vi "运维调试_挥发酚.vi"() -> ()   [LabVIEW 2016, in "挥发酚.lvlib"]
uses:
  <vilib>/Utility/miscctls.llb/LVPointTypeDef.ctl
  <vilib>/ptbypt/NI_PtbyPt.lvlib
panel:
  out "当前步骤:":string
  in  "告警代码":u16
  in  "周期设置":bool
  out "权限等级":string
  in  "参数查询":bool
  in  "平台反控标样校准":enum16{"标液1", "标液2", "标液3"}(ring)
  in  "平台反控校准量程":enum16{"低量程1", "低量程2", "高量程1", "高量程2"}(ring)
  in  "返回 3":bool
  in  "返回 2":bool
  out "单位:":T1(ring)
  out "运行状态":T2 {"数据时间:" format="%<%y/%m/%d %H:%M:%S>T"; "仪器时间:" format="%<%y/%m/%d %H:%M:%S>T"}
  out "模块版本号":string
  in  "布尔":bool
  out "字符串":string
  in  "返回":bool
  in  "设置":bool
  out "集成报警信息":string
  in  "停止":bool
  in  "手动启动":bool
  # "."
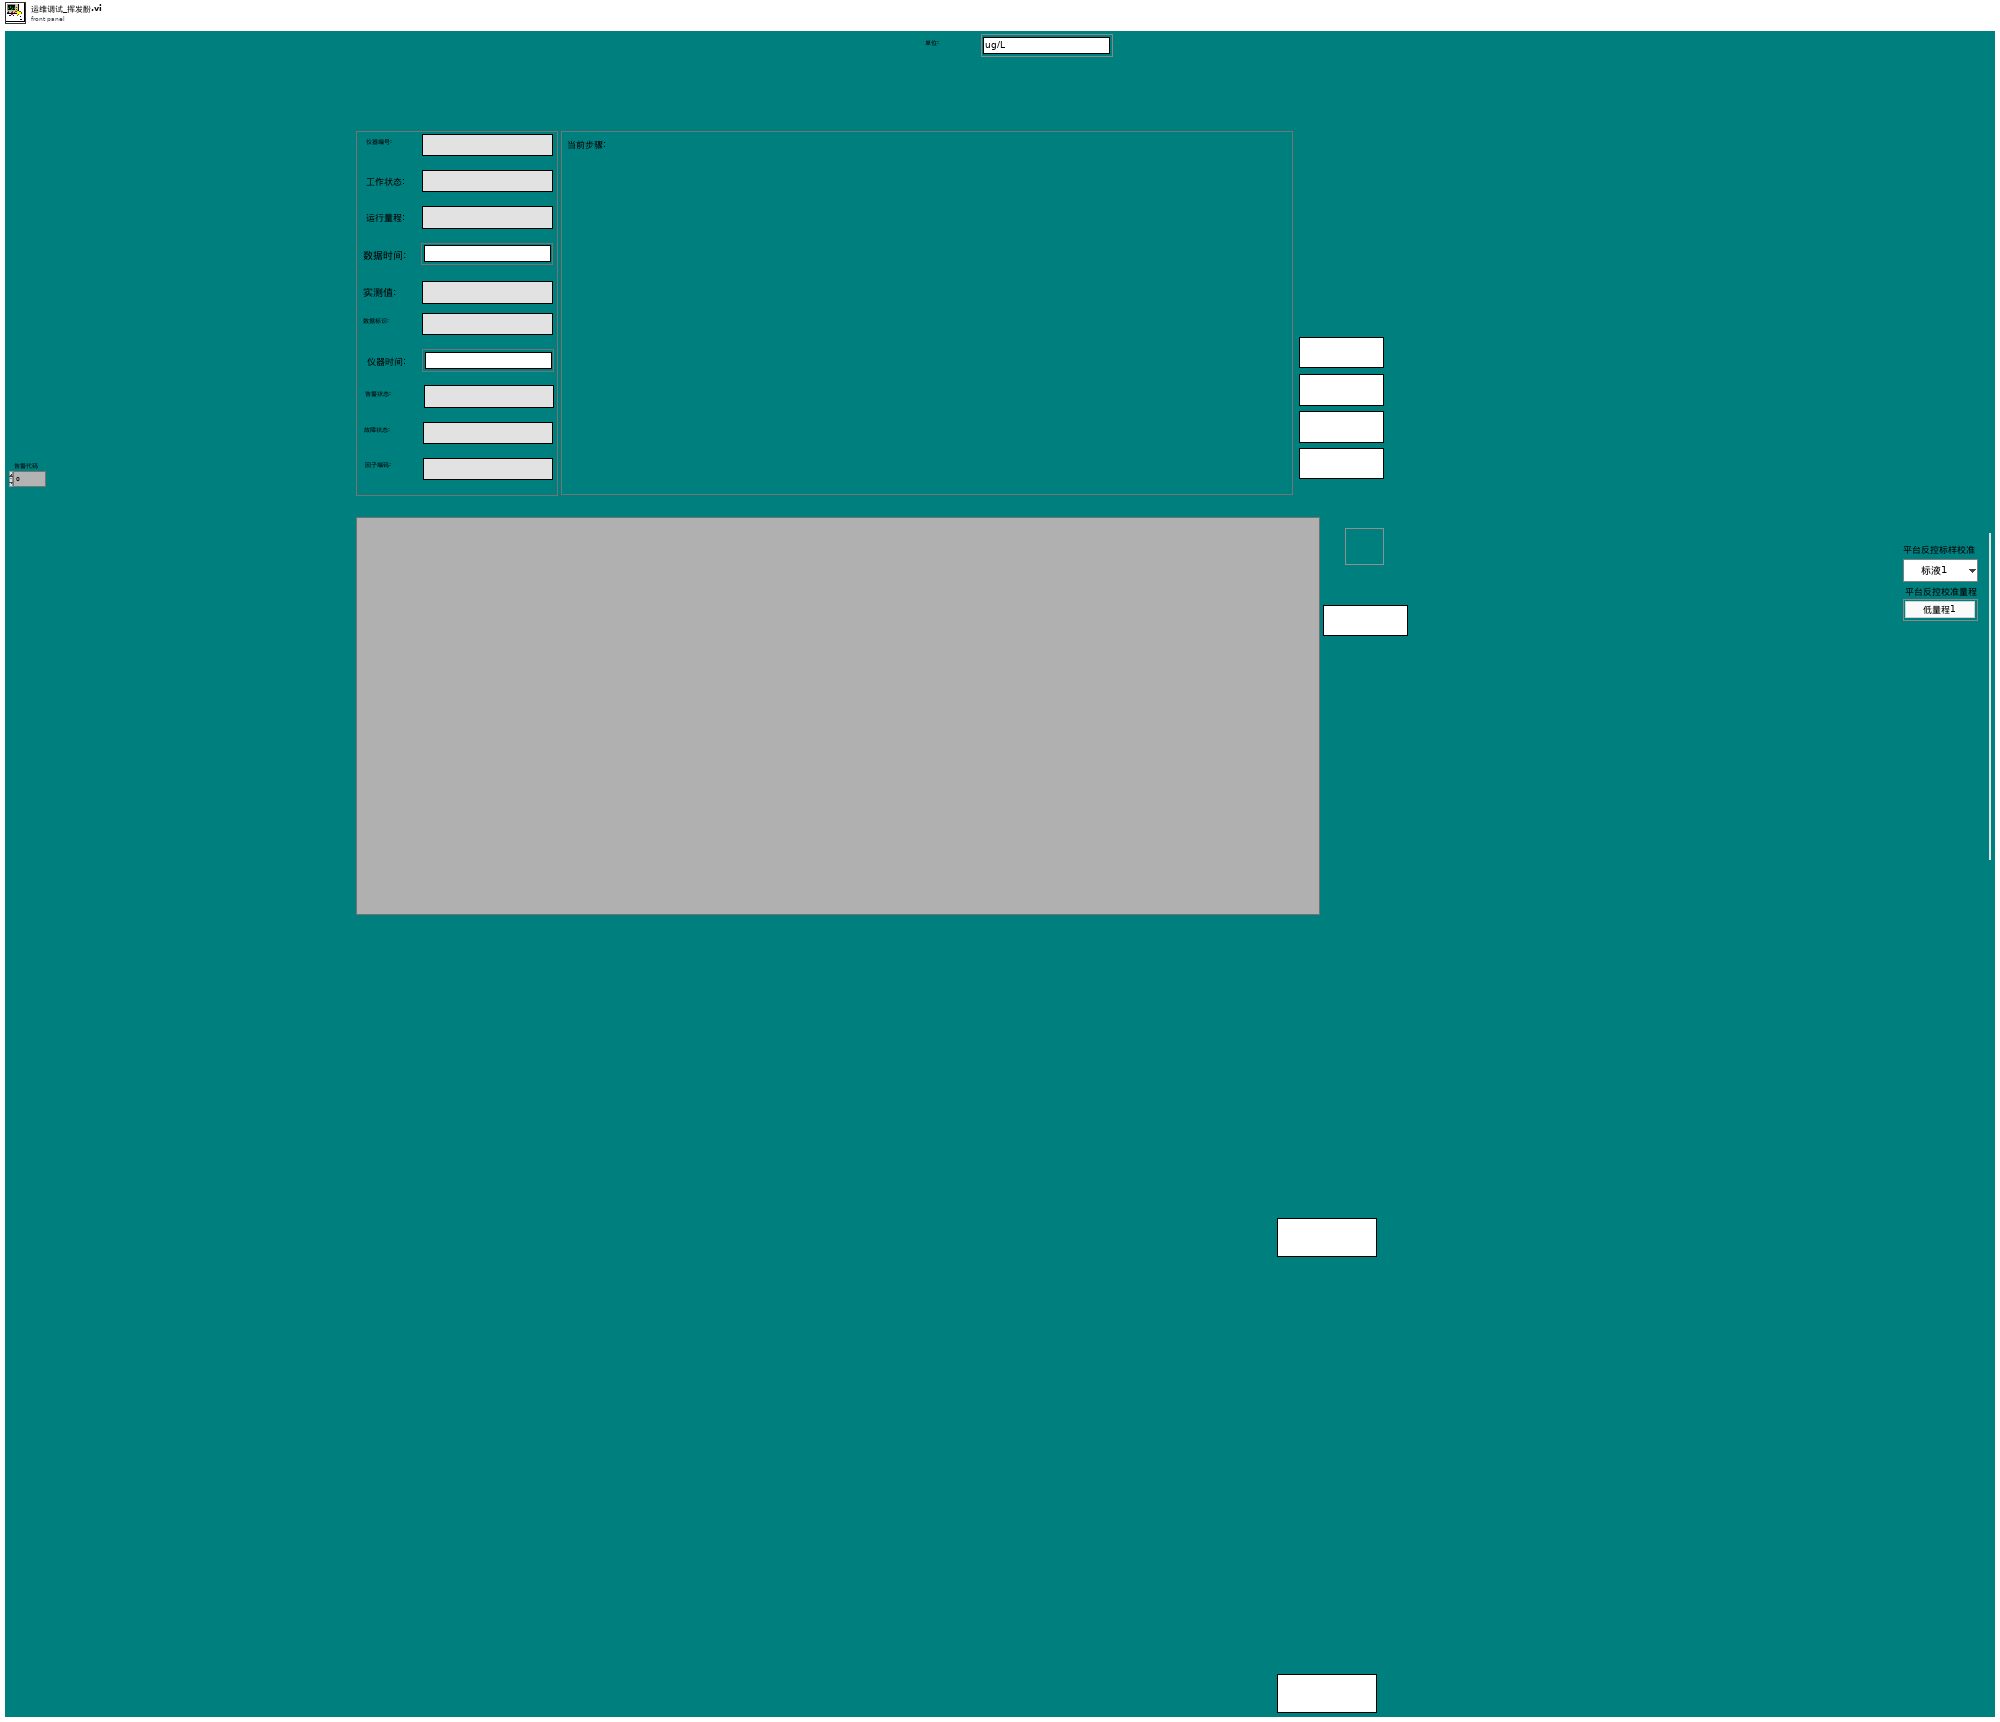
[diagram p1: front panel]
types:
  T1 = enum16{"ug/L", "mg/L", "ppm", "mg/m3", "cm", "ppb", "ug/m3", "%", "nmol/mol", "umol/mol", "MPN/L", "MPN/100ml", "ng/m3", "NTU", "无量纲", "ms/cm", "us/cm", "℃", "mV", "万个/L"}
  T2 = cluster{"仪器编号:":string, "工作状态:":string, "运行量程: ":string, "数据时间:":timestamp, "实测值:":string, "数据标识: ":string, "仪器时间:":timestamp, "告警状态: ":string, "故障状态:  ":string, "因子编码:":string}
  T3 = cluster{"Major":u16, "Minor":u16, "Fix":u16, "Build":u16}
  T4 = typedef "LVPointTypeDef.ctl" = cluster{"Horizontal":i16, "Vertical":i16}
  T5 = cluster{"因子编码":u32, "单位":u16, "标样2参考值":sgl, "水样数据时间":timestamp, "水样实测值":sgl, "水样数据标识":string, "标样2数据时间":timestamp, "标样2实测值":sgl, "标样2数据标识":string, "空白数据时间":timestamp, "空白实测值":sgl, "空白数据标识":string, "零点核查数据时间":timestamp, "零点核查实测值":sgl, "零点核查数据标识":string, "跨度核查数据时间":timestamp, "跨度核查实测值":sgl, "跨度核查数据标识":string, "加标回收数据时间":timestamp, "加标回收实测值":sgl, "加标回收数据标识":string, "平行样数据时间":timestamp, "平行样实测值":sgl, "平行样数据标识":string, "标样1参考值":sgl, "标样1数据时间":timestamp, "标样1实测值":sgl, "标样1数据标识":string, "标样核查数据时间":timestamp, "标样核查实测值":sgl, "标样核查数据标识":string}
  T6 = cluster{"系统时间":timestamp, "工作状态":u16, "测量模式":enum16{"待机", "连续模式", "周期模式", "定点模式", "受控模式", "手动模式"}, "告警代码":u16, "故障代码":u16, "日志代码":u16, "软件版本":u16, "测量间隔":u16, "消解实时温度":dbl, "校准间隔（天）":u16, "校准间隔（时）":u16, "周期测量时间（23_16）":u16, "周期测量时间（15_0）":u16, "清洗周期（次数）":u16, "运行模式":u16, "自动校准状态":u16, "自动清洗状态":u16}
  T7 = cluster{"测量精度":u16, "消解温度":u16, "消解时长":u16, "量程下限":sgl, "量程上限":sgl, "曲线斜率K":sgl, "曲线斜率B":sgl, "标定日期":timestamp, "标液1浓度":sgl, "标液1测量过程值":sgl, "标液2浓度":sgl, "标液2测量过程值":sgl, "标液3浓度":sgl, "标液3测量过程值":sgl, "标液4浓度":sgl, "标液4测量过程值":sgl, "标液5浓度":sgl, "标液5测量过程值":sgl, "线性相关系数":sgl, "试剂余量":u32, "测量滴定值或吸光度":sgl, "标样2校准时间":timestamp, "检出限值":sgl, "校准系数":sgl, "设备系列号":string, "显色温度":u16, "显色时间":u16, "试剂余量1":u16, "试剂余量2":u16, "试剂余量3":u16, "试剂余量4":u16, "试剂余量5":u16, "试剂余量6":u16, "试剂余量7":u16, "试剂余量8":u16, "试剂余量9":u16, "试剂余量10":u16, "当前量程低位":sgl, "当前量程高位":sgl}
  T8 = typedef "Alarm interface.lvlib/报警短信语音交互.ctl" = cluster{"参数":string, "元器件":string, "故障现象":string, "code":string, "platform_alarm_code":string, "solutionList":cluster{"reason":string, "solution":string}[]}
  T9 = enum8{"Enabled", "Disabled", "Disabled and Grayed Out"}
  T10 = enum32{"Bad", "Idle", "Run top level", "Running"}
  T11 = enum16{"空闲", "水样测试", "标样核查", "零点核查", "跨度核查", "空白测试", "平行样测试", "加标回收", "空白校准", "标样校准", "初始化（清洗）"}
  T12 = typedef "TimingControl.lvlib/TimingControl.lvclass/国标控制命令.ctl" = enum16{"启动测量", "标样核查", "零点核查", "跨度核查", "空白测试", "平行样测试", "加标回收", "空白校准", "标样校准", "初始化（清洗）", "停止测试", "仪器重启", "校时", "模式设置", "测量间隔设置"}
  T13 = typedef "TimingControl.lvlib/TimingControl.lvclass/测量参数.ctl" = u16
  T14 = cluster{"时间标识":timestamp, "设备":string, "日志信息":string, "流程参数":string}
  T15 = cluster{"水样数据时间":timestamp, "空白数据时间":timestamp, "零点核查数据时间":timestamp, "跨度核查数据时间":timestamp, "加标回收数据时间":timestamp, "平行样数据时间":timestamp, "标样核查数据时间":timestamp, "标样1数据时间":timestamp, "标样2数据时间":timestamp}
  T16 = cluster{"站号":u16, "量程切换":enum32{"H", "L", "AUTO"}, "控制命令":u16, "模式设置":enum16{"待机", "连续模式", "周期模式", "定点模式", "受控模式", "手动模式"}, "测量间隔":u16}
  T17 = cluster{"跨度值":dbl, "零点标准液浓度":dbl, "跨度标准液浓度":dbl, "标准液标准浓度":dbl, "零点标准液偏差":dbl, "跨度标准液偏差":dbl, "标准液标准偏差":dbl}
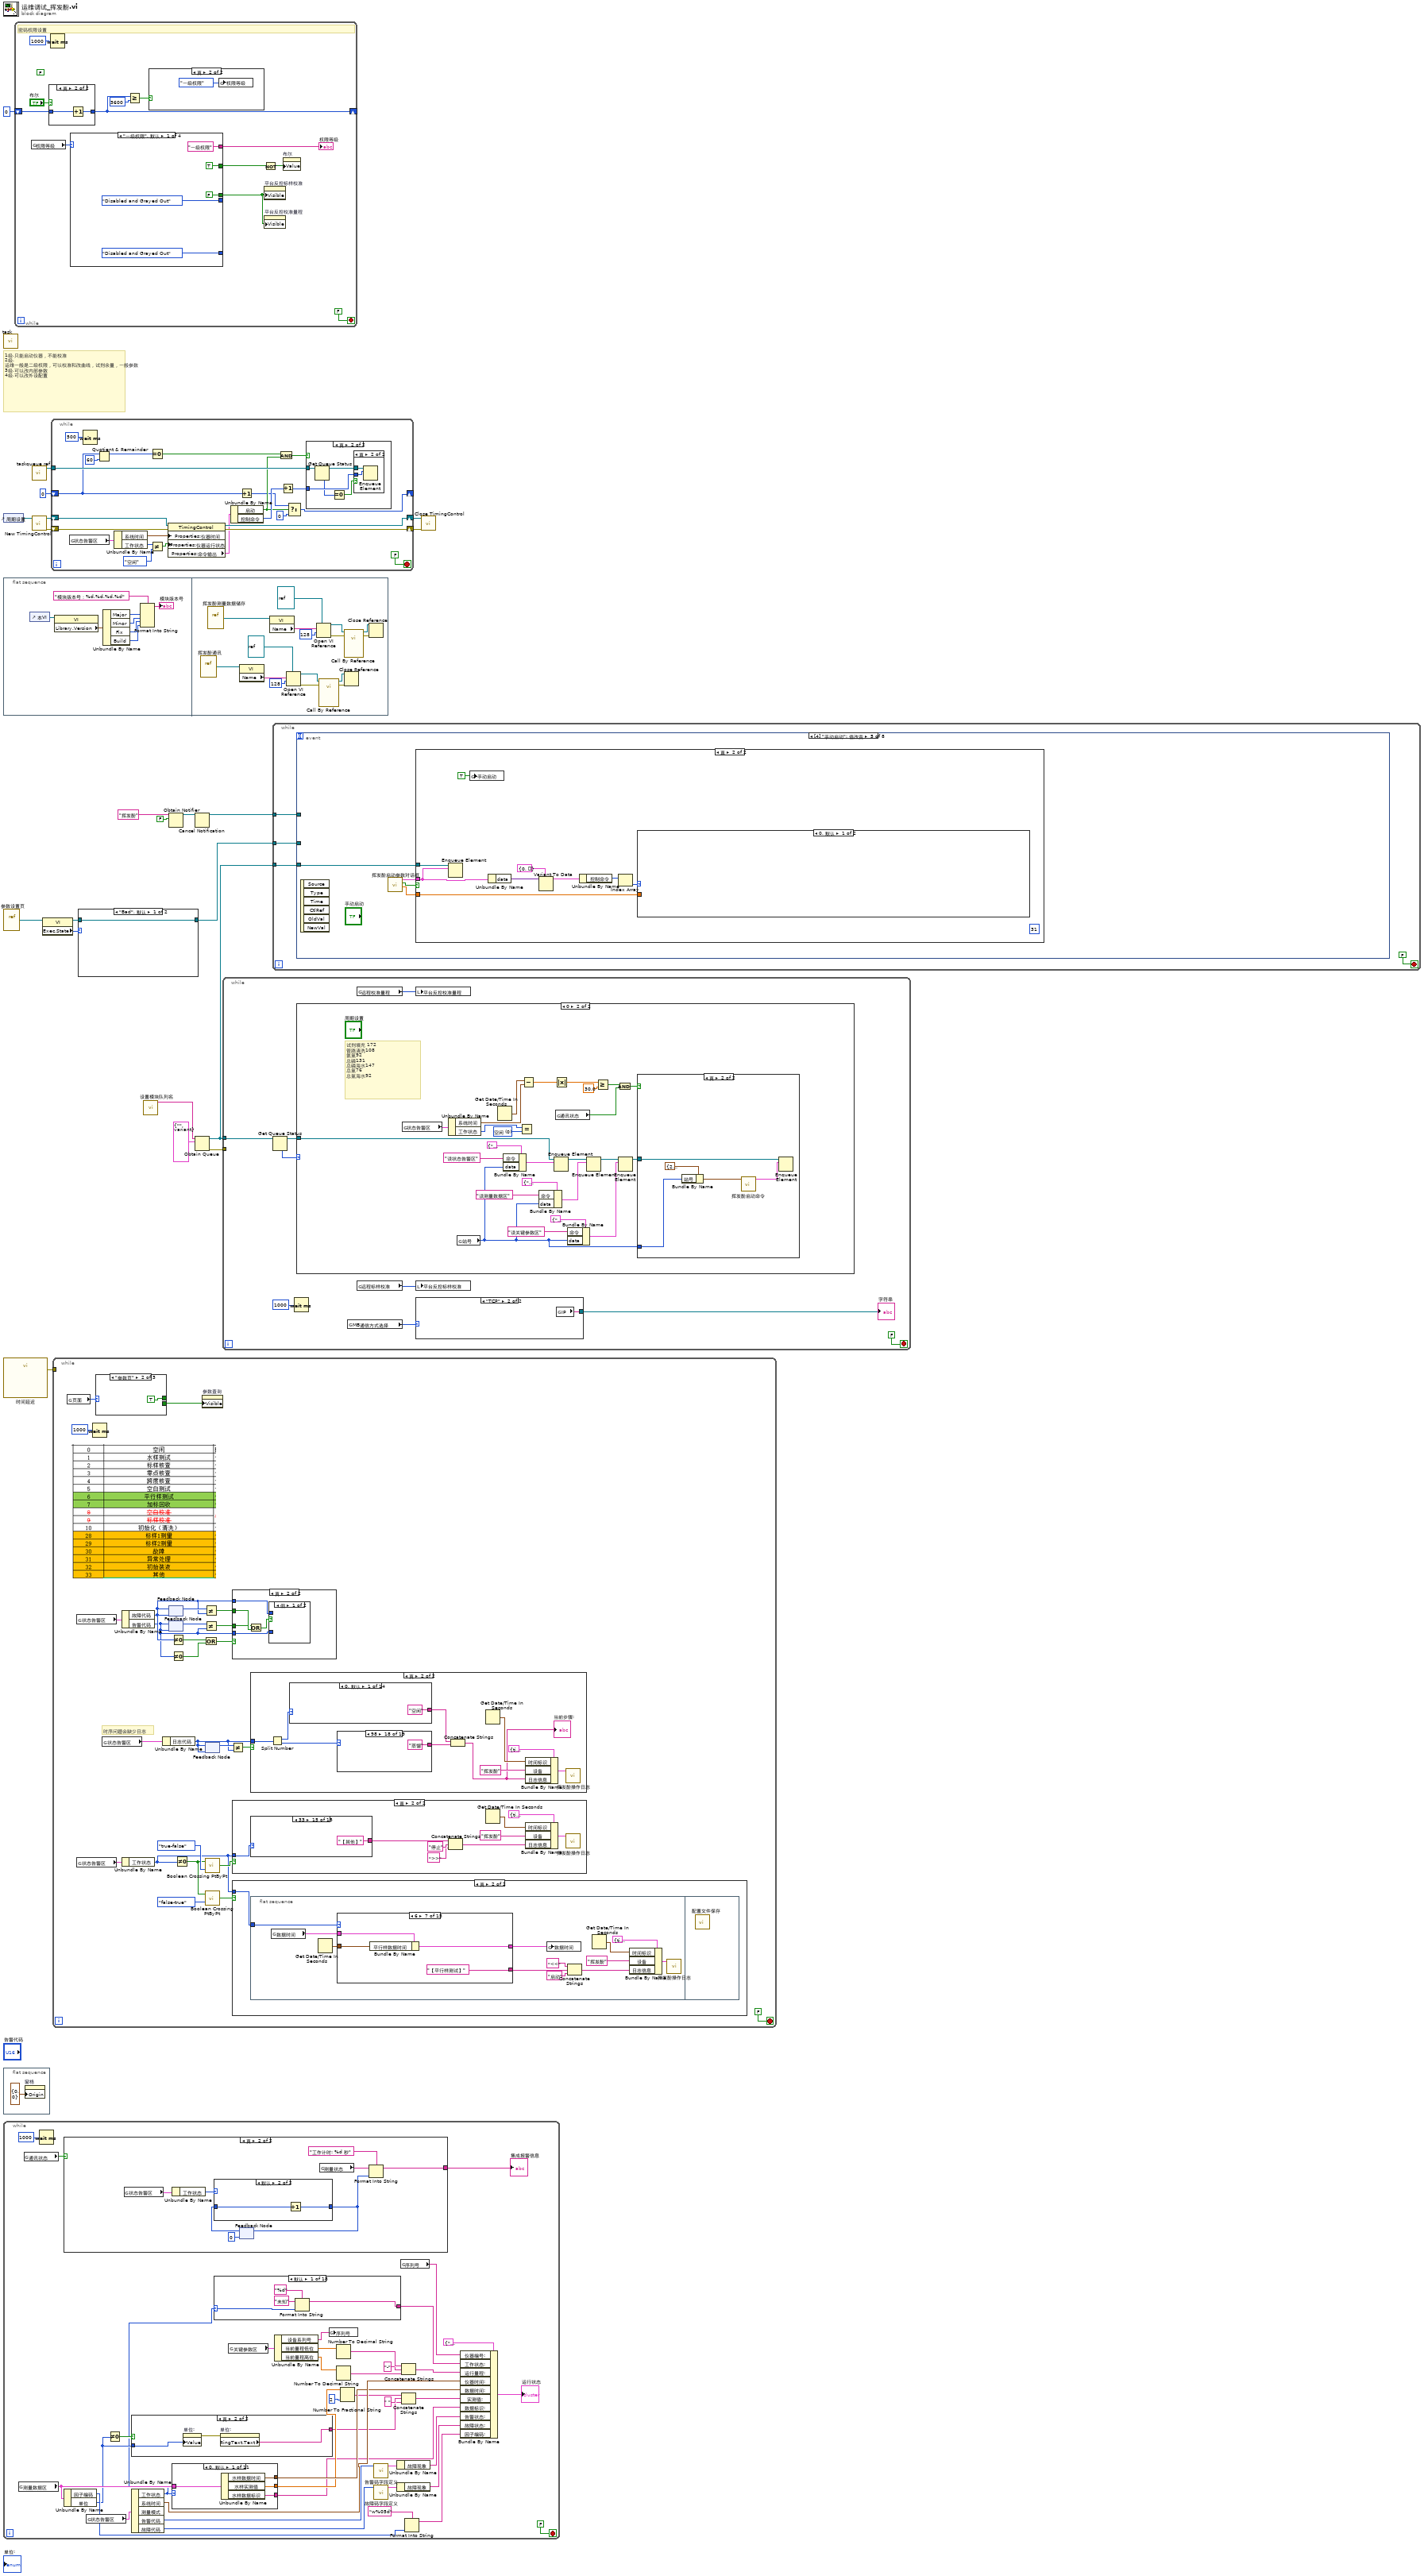
[diagram p0: block diagram]
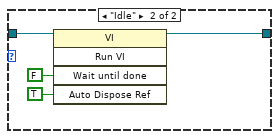
[diagram p2: hidden frame]
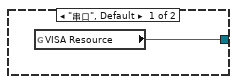
[diagram p5: hidden frame]
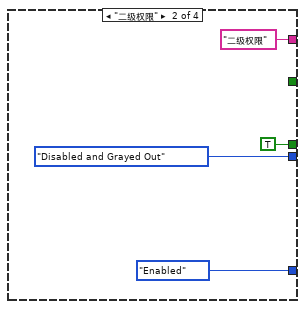
[diagram p8: hidden frame]
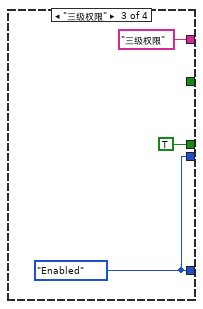
[diagram p9: hidden frame]
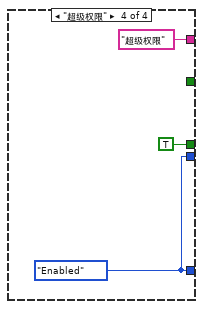
[diagram p10: hidden frame]
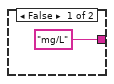
[diagram p13: hidden frame]
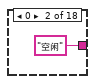
[diagram p14: hidden frame]
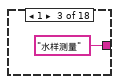
[diagram p15: hidden frame]
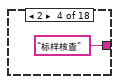
[diagram p16: hidden frame]
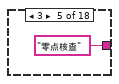
[diagram p17: hidden frame]
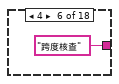
[diagram p18: hidden frame]
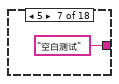
[diagram p19: hidden frame]
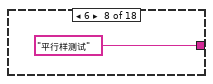
[diagram p20: hidden frame]
diagram:
  # "1级.只能启动仪器，不能校准\n2级.运维一般是二级权限，可以校准和改曲线，试剂余量，一般参数\n3级.可以改内部参数\n4级.可以改外设配置"
  n1 = call "task.vi"() -> ()  [unwired: 12 in]
  n2 = control-ref of="周期设置"() -> (w5:refnum<vi>)
  n3 = flat-sequence {
    frame #0 {
      n4 = control-ref of="本VI"() -> (w29:refnum<vi>)
      n5 = property class="VI"(reference=w29) -> ("Library.Version"=w28:T3)  [unwired: 1 in, 2 out]
      n6 = Unbundle By Name(w28) -> ("Major"=w26:u16, "Minor"=w25:u16, "Fix"=w24:u16, "Build"=w23:u16)
      n7 = Format Into String(format string="模块版本号：%d.%d.%d.%d" ("格式字符串"), w26, w25, w24, w23) -> (resulting string=→"模块版本号":string)  [unwired: 2 in, 1 out]
    }
    frame #1 {
      n8 = vi-ref "挥发酚通讯.vi"() -> (w37:refnum<vi>)
      n9 = vi-ref "挥发酚测量数据储存.vi"() -> (w45:refnum<vi>)
      n10 = property class="VI"(reference=w37) -> ("Name"=w36:string)  [unwired: 1 in, 2 out]
      n11 = property class="VI"(reference=w45) -> ("Name"=w38:string)  [unwired: 1 in, 2 out]
      n12 = Open VI Reference(type specifier VI Refnum (for type only)=refnum<vi> refnum, vi path=w36, options=128 ("选项")) -> (vi reference=w34:refnum<vi>, error out=w32:errorcluster)  [unwired: 3 in]
      n13 = Open VI Reference(type specifier VI Refnum (for type only)=refnum<vi> refnum, vi path=w38, options=128 ("选项")) -> (vi reference=w40:refnum<vi>, error out=w42:errorcluster)  [unwired: 3 in]
      n14 = call-by-ref "?"(reference=w34, error in=w32) -> (reference out=w30:refnum<vi>, error out=w31:errorcluster)  [unwired: 12 in]
      n15 = call-by-ref "?"(reference=w40, error in=w42) -> (reference out=w44:refnum<vi>, error out=w43:errorcluster)  [unwired: 12 in]
      n16 = Close Reference(reference=w30, error in (no error)=w31) -> ()  [unwired: 1 out]
      n17 = Close Reference(reference=w44, error in (no error)=w43) -> ()  [unwired: 1 out]
    }
  }
  n18 = vi-ref "参数设置页.vi"() -> (w12:refnum<vi>)
  n19 = call "时间延迟"() -> ("error out"=w19:errorcluster)  [unwired: 11 in]
  n20 = flat-sequence {
    frame #0 {
      n21 = property on="窗格" class="Pane"("Origin"=T4 {"Horizontal"=0, "Vertical"=0} ("原点")) -> ()  [unwired: 2 in, 2 out]
    }
  }
  n22 = while {
    stop <- FALSE stop-if-true
    n23 = global read "VAR挥发酚全局变量.vi" "测量数据区"() -> (w80:T5)
    n24 = global read "VAR挥发酚全局变量.vi" "通讯状态"() -> (w83:bool)
    n25 = Wait (ms)(milliseconds to wait=u32 1000 ("等待时间（毫秒）")) -> ()  [unwired: 1 out]
    n26 = case shown="真" w83 {
      tunnel: ["通讯异常" ("集成报警信息") w157] -> w82
      frame False {
      }
      frame True {
        n27 = global read "VAR挥发酚全局变量.vi" "状态告警区"() -> (w163:T6)
        n28 = Unbundle By Name(w163) -> ("工作状态"=w162:u16)
        n29 = feedback #1(0) -> (w160:i32)
        n30 = case shown="默认" w162 {
          tunnel: w160 -> [_ w165]
          tunnel: [_ w164] -> w158
          frame 0 {
          }
          frame Default {
            n31 = Increment(x=w165) -> (x+1=w164:i32)
          }
        }
        n32 = feedback-in #1(w158) -> ()
        n33 = global read "VAR挥发酚全局变量.vi" "测量状态"() -> (w156:string)
        n34 = Format Into String(format string="工作计时: %d 秒" ("格式字符串"), initial string=w156, w158) -> (resulting string=w157:string)  [unwired: 1 in, 1 out]
      }
    }
    "集成报警信息" <- w82
    n35 = Unbundle By Name(w80) -> ("因子编码"=w63:u32, "单位"=w60:u16)
    n36 = global read "VAR挥发酚全局变量.vi" "状态告警区"() -> (w81:T6)
    n37 = Not Equal To 0?(x=w60) -> (x != 0?=w61:bool)
    n38 = case shown="真" w61 {
      tunnel: ["mg/L" ("RingText.Text") w88] -> w65
      tunnel: w60 -> [_ w87]
      frame False {
      }
      frame True {
        n39 = property on="单位:" class="Enum (严格)"("Value"=w87) -> (error out=w89:errorcluster)  [unwired: 2 in, 1 out]
        n40 = property on="单位:" class="Enum (严格)"(error in=w89) -> ("RingText.Text"=w88:string)  [unwired: 1 in, 2 out]
      }
    }
    n41 = Unbundle By Name(w81) -> ("工作状态"=w55:u16, "系统时间"=w77:timestamp, "告警代码"=w67:u16, "故障代码"=w66:u16)  [unwired: 1 out]
    n42 = case shown="0, 默认" w55 {
      tunnel: [w114 w118 w122 w126 w130 w134 w138 w142 w145 w149 w154] -> w74
      tunnel: [w112 w117 w121 w125 w129 w133 w136 w141 w144 w148 w153] -> w69
      tunnel: [w111 w116 w120 w124 w128 w132 w135 w140 w143 w147 w152] -> w68
      tunnel: w80 -> [w113 w115 w119 w123 w127 w131 w137 w139 w146 w150 w151]
      frame 0, Default {
        n43 = Unbundle By Name(w113) -> ("水样数据时间"=w114:timestamp, "水样实测值"=w112:sgl, "水样数据标识"=w111:string)
      }
      frame 1 {
        n44 = Unbundle By Name(w115) -> ("水样数据时间"=w118:timestamp, "水样实测值"=w117:sgl, "水样数据标识"=w116:string)
      }
      frame 2 {
        n45 = Unbundle By Name(w119) -> ("标样核查数据时间"=w122:timestamp, "标样核查实测值"=w121:sgl, "标样核查数据标识"=w120:string)
      }
      frame 3 {
        n46 = Unbundle By Name(w123) -> ("零点核查数据时间"=w126:timestamp, "零点核查实测值"=w125:sgl, "零点核查数据标识"=w124:string)
      }
      frame 4 {
        n47 = Unbundle By Name(w127) -> ("跨度核查数据时间"=w130:timestamp, "跨度核查实测值"=w129:sgl, "跨度核查数据标识"=w128:string)
      }
      frame 5 {
        n48 = Unbundle By Name(w131) -> ("空白数据时间"=w134:timestamp, "空白实测值"=w133:sgl, "空白数据标识"=w132:string)
      }
      frame 6 {
        n49 = Unbundle By Name(w137) -> ("平行样数据时间"=w138:timestamp, "平行样实测值"=w136:sgl, "平行样数据标识"=w135:string)
      }
      frame 7 {
        n50 = Unbundle By Name(w139) -> ("加标回收数据时间"=w142:timestamp, "加标回收实测值"=w141:sgl, "加标回收数据标识"=w140:string)
      }
      frame 28 {
        n51 = Unbundle By Name(w146) -> ("标样1数据时间"=w145:timestamp, "标样1实测值"=w144:sgl, "标样1数据标识"=w143:string)
      }
      frame 29 {
        n52 = Unbundle By Name(w150) -> ("标样2数据时间"=w149:timestamp, "标样2实测值"=w148:sgl, "标样2数据标识"=w147:string)
      }
      frame 10 {
        n53 = Unbundle By Name(w151) -> ("水样数据时间"=w154:timestamp, "水样实测值"=w153:sgl, "水样数据标识"=w152:string)
      }
    }
    n54 = case shown="默认" w55 {
      selector: w55 -> [w90 _ _ _ _ _ _ _ _ _ _ _ _ _ _ _ _ _]
      tunnel: [w91 "空闲" ("工作状态") "水样测量" ("工作状态") "标样核查" ("工作状态") "零点核查" ("工作状态") "跨度核查" ("工作状态") "空白测试" ("工作状态") "平行样测试" ("工作状态") "加标回收" ("工作状态") "空白校准" ("工作状态") "标样校准" ("工作状态") "初始化" ("工作状态") "标样1测量" ("工作状态") "标样2测量" ("工作状态") "故障" ("工作状态") "异常处理" ("工作状态") "初始装液" ("工作状态") "其他" ("工作状态")] -> w78
      frame Default {
        n55 = Format Into String(format string="%d" ("格式字符串"), initial string="未知" ("工作状态"), w90) -> (resulting string=w91:string)  [unwired: 1 in, 1 out]
      }
      frame 0 {
      }
      frame 1 {
      }
      frame 2 {
      }
      frame 3 {
      }
      frame 4 {
      }
      frame 5 {
      }
      frame 6 {
      }
      frame 7 {
      }
      frame 8 {
      }
      frame 9 {
      }
      frame 10 {
      }
      frame 28 {
      }
      frame 29 {
      }
      frame 30 {
      }
      frame 31 {
      }
      frame 32 {
      }
      frame 33 {
      }
    }
    n56 = global read "VAR挥发酚全局变量.vi" "关键参数区"() -> (w54:T7)
    n57 = Unbundle By Name(w54) -> ("设备系列号"=w53:string, "当前量程低位"=w52:sgl, "当前量程高位"=w49:sgl)
    n58 = global write "VAR挥发酚全局变量.vi" "序列号"(w53) -> ()
    n59 = Number To Decimal String(number=w52) -> (decimal integer string=w51:string)  [unwired: 1 in]
    n60 = Number To Decimal String(number=w49) -> (decimal integer string=w48:string)  [unwired: 1 in]
    n61 = Number To Fractional String(number=w69, precision (6)=i16 2 ("精度(6)")) -> (F-format string=w72:string)  [unwired: 2 in]
    n62 = call "告警码字段定义.vi"("告警代码"=w67) -> ("data"=w59:T8)  [unwired: 10 in]
    n63 = call "故障码字段定义.vi"("故障代码"=w66) -> ("data"=w58:T8)  [unwired: 10 in]
    n64 = Unbundle By Name(w59) -> ("故障现象"=w56:string)
    n65 = Unbundle By Name(w58) -> ("故障现象"=w57:string)
    n66 = global read "VAR挥发酚全局变量.vi" "序列号"() -> (w79:string)
    n67 = Concatenate Strings(w51, "-" ("字符串"), w48) -> (w47:string)
    n68 = Concatenate Strings(w72, " " ("字符串"), w65) -> (w70:string)
    n69 = Format Into String(format string="w%05d" ("格式字符串"), w63) -> (resulting string=w62:string)  [unwired: 2 in, 1 out]
    n70 = Bundle By Name(cluster=T2 {"仪器编号:"="", "工作状态:"="", "运行量程: "="", "数据时间:"=timestamp(0 s since 1904-01-01), "实测值:"="", "数据标识: "="", "仪器时间:"=timestamp(0 s since 1904-01-01), "告警状态: "="", "故障状态:  "="", "因子编码:"=""} ("运行状态"), "仪器编号:"=w79, "工作状态:"=w78, "运行量程:"=w47, "仪器时间:"=w77, "数据时间:"=w74, "实测值:"=w70, "数据标识:"=w68, "告警状态:"=w56, "故障状态:"=w57, "因子编码:"=w62) -> (→"运行状态":T2)
  }
  n71 = while {
    shift-right: [w174] -> _
    shift-left: u32 0 ("等待时间（毫秒）") -> [w175]
    stop <- FALSE stop-if-true
    (unwired) FALSE ("可见")
    # "密码权限设置"
    n72 = global read "VAR挥发酚全局变量.vi" "权限等级"() -> (w171:enum16{"一级权限", "二级权限", "三级权限", "超级权限"})
    n73 = case shown="真" "布尔" {
      tunnel: w175 -> [_ w195]
      tunnel: [_ w194] -> w174
      frame False {
      }
      frame True {
        n74 = Increment(x=w195) -> (x+1=w194:u32)
      }
    }
    n75 = Wait (ms)(milliseconds to wait=u32 1000 ("等待时间（毫秒）")) -> ()  [unwired: 1 out]
    n76 = case shown="\"一级权限\", 默认" w171 {
      tunnel: [T9."Disabled and Grayed Out" ("f") T9."Enabled" ("禁用") w189 w192] -> _
      tunnel: [T9."Disabled and Grayed Out" ("f") T9."Disabled and Grayed Out" ("f") w189 w192] -> _
      tunnel: [FALSE ("可见") TRUE ("可见") TRUE ("可见") TRUE ("可见")] -> w170
      tunnel: ["一级权限" "二级权限" "三级权限" "超级权限"] -> w169
      tunnel: [TRUE _ _ _] -> w168
      frame "一级权限", Default {
      }
      frame "二级权限" {
      }
      frame "三级权限" {
        w189 = T9."Enabled" ("禁用")
      }
      frame "超级权限" {
        w192 = T9."Enabled" ("禁用")
      }
    }
    "权限等级" <- w169
    n77 = Greater Or Equal?(x=w174, y=u32 3600) -> (x >= y?=w172:bool)
    n78 = case shown="真" w172 {
      frame False {
      }
      frame True {
        n79 = global write "VAR挥发酚全局变量.vi" "权限等级"(enum16{"一级权限", "二级权限", "三级权限", "超级权限"}."一级权限" ("权限等级")) -> ()
      }
    }
    n80 = Not(x=w168) -> (.not. x?=w166:bool)
    n81 = property on="平台反控标样校准" class="Enum (严格)"("Visible"=w170) -> ()  [unwired: 2 in, 2 out]
    n82 = property on="平台反控校准量程" class="Enum (严格)"("Visible"=w170) -> ()  [unwired: 2 in, 2 out]
    n83 = property on="布尔" class="Bool (严格)"("Value"=w166) -> ()  [unwired: 2 in, 2 out]
  }
  n84 = call "taskqueue ref.vi"() -> ("队列输出"=w8:refnum<queue>)  [unwired: 10 in, 1 out]
  n85 = call "New TimingControl.vi"("Reference"=w5) -> ("error out"=w3:errorcluster, "TimingControl out"=w4:refnum<class "TimingControl.lvclass">)  [unwired: 9 in]
  n86 = property class="VI"(reference=w12) -> (reference out=w10:refnum<vi>, "Exec.State"=w11:T10)  [unwired: 1 in, 1 out]
  n87 = while {
    tunnel: w8 -> [w215]
    shift-right: [w205] -> _
    shift-left: u32 0 ("等待时间（毫秒）") -> [w206]
    shift-right: [w200] -> w2
    shift-left: w4 -> [w202]
    shift-right: [w199] -> w1
    shift-left: w3 -> [w201]
    stop <- FALSE stop-if-true
    n88 = global read "VAR挥发酚全局变量.vi" "状态告警区"() -> (w217:T6)
    n89 = Wait (ms)(milliseconds to wait=u32 500 ("等待时间（毫秒）")) -> ()  [unwired: 1 out]
    n90 = Quotient & Remainder(x=w206, y=u32 60) -> (x-y*floor(x/y)=w203:u32)  [unwired: 1 out]
    n91 = Unbundle By Name(w217) -> ("系统时间"=w197:timestamp, "工作状态"=w210:u16)
    n92 = Equal To 0?(x=w203) -> (x = 0?=w212:bool)
    n93 = Not Equal?(x=w210, y=T11."空闲") -> (x != y?=w196:bool)
    n94 = property class="TimingControl"(reference=w202, error in=w201, "Properties:仪器时间"=w197, "Properties:仪器运行状态"=w196) -> (reference out=w200:refnum<class "TimingControl.lvclass">, error out=w199:errorcluster, "Properties:命令输出"=w198:cluster{"启动":bool, "控制命令":T12, "测量参数":T13})
    n95 = Unbundle By Name(w198) -> ("启动"=w209:bool, "控制命令"=w214:T12)
    n96 = Increment(x=w206) -> (x+1=w208:u32)
    n97 = And(x=w212, y=w209) -> (x .and. y?=w211:bool)
    n98 = Increment(x=w214) -> (x+1=w213:T12)
    n99 = Select(t=w208, s=w209, f=u32 0) -> (s? t:f=w205:u32)
    n100 = case shown="真" w211 {
      tunnel: w215 -> [_ w224]
      tunnel: w213 -> [_ w223]
      frame False {
      }
      frame True {
        n101 = Get Queue Status(queue=w224) -> (queue out=w222:refnum<queue>, # elements in queue=w221:i32)  [unwired: 2 in, 6 out]
        n102 = Equal To 0?(x=w221) -> (x = 0?=w220:bool)
        n103 = case shown="真" w220 {
          tunnel: w223 -> [_ w226]
          tunnel: w222 -> [_ w225]
          frame False {
          }
          frame True {
            n104 = Enqueue Element(queue=w225, element=w226) -> ()  [unwired: 2 in, 3 out]
          }
        }
      }
    }
  }
  n105 = while {
    tunnel: w19 -> [_]
    stop <- FALSE stop-if-true
    # "时序问题会缺少日志"
    n106 = global read "VAR挥发酚全局变量.vi" "页面"() -> (w232:enum16{"主页", "参数页", "校准页"})
    n107 = global read "VAR挥发酚全局变量.vi" "状态告警区"() -> (w249:T6)
    n108 = global read "VAR挥发酚全局变量.vi" "状态告警区"() -> (w246:T6)
    n109 = Wait (ms)(milliseconds to wait=u32 1000 ("等待时间（毫秒）")) -> ()  [unwired: 1 out]
    n110 = case shown="\"参数页\"" w232 {
      tunnel: [_ _ TRUE ("可见")] -> w231
      tunnel: [_ TRUE ("可见") _] -> _
      frame "主页", Default {
      }
      frame "参数页" {
      }
      frame "校准页" {
      }
    }
    n111 = global read "VAR挥发酚全局变量.vi" "状态告警区"() -> (w230:T6)
    n112 = Unbundle By Name(w249) -> ("故障代码"=w235:u16, "告警代码"=w234:u16)
    n113 = Unbundle By Name(w246) -> ("工作状态"=w240:u16)
    n114 = Unbundle By Name(w230) -> ("日志代码"=w227:u16)
    n115 = feedback #2(w235) -> (w247:u16)
    n116 = feedback-in #2(w235) -> ()
    n117 = feedback #3(w234) -> (w239:u16)
    n118 = feedback-in #3(w234) -> ()
    n119 = Not Equal To 0?(x=w235) -> (x != 0?=w237:bool)
    n120 = Not Equal To 0?(x=w234) -> (x != 0?=w236:bool)
    n121 = Not Equal To 0?(x=w240) -> (x != 0?=w242:bool)
    n122 = property on="参数查询" class="Bool"("Visible"=w231) -> ()  [unwired: 2 in, 2 out]
    n123 = Not Equal?(x=w247, y=w235) -> (x != y?=w248:bool)
    n124 = Not Equal?(x=w239, y=w234) -> (x != y?=w238:bool)
    n125 = Or(x=w237, y=w236) -> (x .or. y?=w233:bool)
    n126 = feedback #4(w227) -> (w229:u16)
    n127 = feedback-in #4(w227) -> ()
    n128 = call <vilib>:"Boolean Crossing PtByPt.vi"("direction"=enum16{"either", "false-true", "true-false"}."true-false", "input"=w242) -> ("crossing"=w241:bool)  [unwired: 1 in]
    n129 = call <vilib>:"Boolean Crossing PtByPt.vi"("direction"=enum16{"either", "false-true", "true-false"}."false-true", "input"=w242) -> ("crossing"=w244:bool)  [unwired: 1 in]
    n130 = Not Equal?(x=w229, y=w227) -> (x != y?=w228:bool)
    n131 = case shown="真" w233 {
      tunnel: w248 -> [_ w384]
      tunnel: w238 -> [_ w382]
      tunnel: w234 -> [_ w381]
      tunnel: w235 -> [_ w380]
      frame False {
      }
      frame True {
        n132 = Or(x=w382, y=w384) -> (x .or. y?=w383:bool)
        n133 = case shown="假" w383 {
          tunnel: w380 -> [_ _]
          tunnel: w381 -> [_ _]
          frame False {
          }
          frame True {
          }
        }
      }
    }
    n134 = case shown="真" w241 {
      tunnel: w240 -> [_ w298]
      frame False {
      }
      frame True {
        n135 = case shown="33" w298 {
          tunnel: [_ "【水样测试】" ("字符串") "【标样核查】" ("字符串") "【零点核查】" ("字符串") "【跨度核查】" ("字符串") "【空白测试】" ("字符串") "【平行样测试】" ("字符串") "【加标回收】" ("字符串") "【初始化(清洗)】" ("字符串") "【标样1校准】" ("字符串") "【标样2校准】" ("字符串") "【故障】" ("字符串") "【异常处理】" ("字符串") "【初始装液】" ("字符串") "【其他】" ("字符串")] -> w297
          frame 0, Default {
          }
          frame 1 {
          }
          frame 2 {
          }
          frame 3 {
          }
          frame 4 {
          }
          frame 5 {
          }
          frame 6 {
          }
          frame 7 {
          }
          frame 10 {
          }
          frame 28 {
          }
          frame 29 {
          }
          frame 30 {
          }
          frame 31 {
          }
          frame 32 {
          }
          frame 33 {
          }
        }
        n136 = Concatenate Strings(w297, "停止" ("字符串"), ">>" ("字符串")) -> (w302:string)
        n137 = Get Date/Time In Seconds() -> (seconds since 1Jan1904=w304:timestamp)
        n138 = Bundle By Name(cluster=T14 {"时间标识"=timestamp(0 s since 1904-01-01), "设备"="", "日志信息"="", "流程参数"=""} ("data in"), "时间标识"=w304, "设备"="挥发酚" ("table输入"), "日志信息"=w302) -> (w303:T14)
        n139 = call "挥发酚操作日志.vi"("data in"=w303) -> ()  [unwired: 11 in]
      }
    }
    n140 = case shown="真" w244 {
      tunnel: w240 -> [_ w320]
      frame False {
      }
      frame True {
        n141 = flat-sequence {
          tunnel: w320 -> [w329]
          frame #0 {
            n142 = global read "挥发酚断电保存全局变量.vi" "数据时间"() -> (w323:T15)
            n143 = Get Date/Time In Seconds() -> (seconds since 1Jan1904=w322:timestamp)
            n144 = case shown="6" w329 {
              tunnel: [_ "【水样测试】" ("字符串") "【标样核查】" ("字符串") "【零点核查】" ("字符串") "【跨度核查】" ("字符串") "【空白测试】" ("字符串") "【平行样测试】" ("字符串") "【加标回收】" ("字符串") "【初始化(清洗)】" ("字符串") "【标样1校准】" ("字符串") "【标样2校准】" ("字符串") "【故障】" ("字符串") "【异常处理】" ("字符串") "【初始装液】" ("字符串") "【其他】" ("字符串")] -> w328
              tunnel: w323 -> [w333 w336 w340 w344 w348 w352 w356 w360 w362 w366 w370 w372 w374 w376 w378]
              tunnel: w322 -> [_ w335 w339 w343 w347 w351 w355 w359 _ w365 w369 _ _ _ _]
              tunnel: [w333 w334 w338 w342 w346 w350 w354 w358 w362 w364 w368 w372 w374 w376 w378] -> w321
              frame 0, Default {
              }
              frame 1 {
                n145 = Bundle By Name(cluster=w336, "水样数据时间"=w335) -> (w334:T15)
              }
              frame 2 {
                n146 = Bundle By Name(cluster=w340, "标样核查数据时间"=w339) -> (w338:T15)
              }
              frame 3 {
                n147 = Bundle By Name(cluster=w344, "零点核查数据时间"=w343) -> (w342:T15)
              }
              frame 4 {
                n148 = Bundle By Name(cluster=w348, "跨度核查数据时间"=w347) -> (w346:T15)
              }
              frame 5 {
                n149 = Bundle By Name(cluster=w352, "空白数据时间"=w351) -> (w350:T15)
              }
              frame 6 {
                n150 = Bundle By Name(cluster=w356, "平行样数据时间"=w355) -> (w354:T15)
              }
              frame 7 {
                n151 = Bundle By Name(cluster=w360, "加标回收数据时间"=w359) -> (w358:T15)
              }
              frame 10 {
              }
              frame 28 {
                n152 = Bundle By Name(cluster=w366, "标样1数据时间"=w365) -> (w364:T15)
              }
              frame 29 {
                n153 = Bundle By Name(cluster=w370, "标样2数据时间"=w369) -> (w368:T15)
              }
              frame 30 {
              }
              frame 31 {
              }
              frame 32 {
              }
              frame 33 {
              }
            }
            n154 = global write "挥发酚断电保存全局变量.vi" "数据时间"(w321) -> ()
            n155 = Concatenate Strings("<<" ("字符串"), w328, "启动" ("字符串")) -> (w327:string)
            n156 = Get Date/Time In Seconds() -> (seconds since 1Jan1904=w331:timestamp)
            n157 = Bundle By Name(cluster=T14 {"时间标识"=timestamp(0 s since 1904-01-01), "设备"="", "日志信息"="", "流程参数"=""} ("data in"), "时间标识"=w331, "设备"="挥发酚" ("table输入"), "日志信息"=w327) -> (w330:T14)
            n158 = call "挥发酚操作日志.vi"("data in"=w330) -> ()  [unwired: 11 in]
          }
          frame #1 {
            n159 = call "配置文件保存.vi"() -> ()  [unwired: 12 in]
          }
        }
      }
    }
    n160 = case shown="真" w228 {
      tunnel: w227 -> [_ w257]
      frame False {
      }
      frame True {
        n161 = Split Number(x=w257) -> (hi(x)=w256:u8, lo(x)=w254:u8)
        n162 = case shown="0, 默认" w256 {
          tunnel: ["空闲" "水样测量" "仪表清洗" "标样1测量" "零样测量" "管路冲洗" "初始装液" "异常处理" "零点核查" "标定" "跨度核查" "标样核查" "加标回收" "平行样测量"] -> w255
          frame 0, Default {
          }
          frame 1 {
          }
          frame 4 {
          }
          frame 5 {
          }
          frame 6 {
          }
          frame 7 {
          }
          frame 8 {
          }
          frame 10 {
          }
          frame 14 {
          }
          frame 16 {
          }
          frame 17 {
          }
          frame 18 {
          }
          frame 19 {
          }
          frame 20 {
          }
        }
        n163 = case shown="98" w254 {
          tunnel: ["" "润洗" "排液" "显色" "读取光强" "清洗" "初始化" "进样品" "进零样" "排空" "进标样" "准备" "进试剂" "静置" "结束" "启动蒸馏" "停止蒸馏" "蒸馏" "其他"] -> w253
          frame 0, Default {
          }
          frame 1 {
          }
          frame 4 {
          }
          frame 7 {
          }
          frame 8 {
          }
          frame 9 {
          }
          frame 10 {
          }
          frame 11 {
          }
          frame 15 {
          }
          frame 16 {
          }
          frame 17 {
          }
          frame 19 {
          }
          frame 21 {
          }
          frame 29 {
          }
          frame 34 {
          }
          frame 96 {
          }
          frame 97 {
          }
          frame 98 {
          }
          frame 99 {
          }
        }
        n164 = Concatenate Strings(w255, w253) -> (w252:string)
        "当前步骤:" <- w252
        n165 = Get Date/Time In Seconds() -> (seconds since 1Jan1904=w259:timestamp)
        n166 = Bundle By Name(cluster=T14 {"时间标识"=timestamp(0 s since 1904-01-01), "设备"="", "日志信息"="", "流程参数"=""} ("data in"), "时间标识"=w259, "设备"="挥发酚" ("table输入"), "日志信息"=w252) -> (w261:T14)
        n167 = call "挥发酚操作日志.vi"("data in"=w261) -> ()  [unwired: 11 in]
      }
    }
  }
  n168 = case shown="\"Bad\", 默认" w11 {
    tunnel: w10 -> [w385 w389]
    tunnel: [w385 w386] -> w9
    frame "Bad", Default {
    }
    frame "Idle" {
      n169 = invoke class="VI" method="Run VI"(reference=w389, "Wait until done"=FALSE ("结束前等待"), "Auto Dispose Ref"=TRUE ("自动销毁引用")) -> (reference out=w386:refnum<vi>)  [unwired: 2 in, 4 out]
    }
  }
  n170 = call "设置模块队列名.vi"() -> ("Msg"=w6:string)  [unwired: 11 in]
  n171 = Obtain Notifier(name (unnamed)="挥发酚" ("名称（未命名）"), notification data type=FALSE) -> (notifier out=w16:refnum<notifier>)  [unwired: 2 in, 2 out]
  n172 = Cancel Notification(0:w16) -> (8:w15:refnum<notifier>)  [unwired: 1 in, 2 out]
  n173 = Obtain Queue(name (unnamed)=w6, element data type=cluster{"命令":string, "data":variant} {"命令"="", "data"=variant}) -> (queue out=w13:refnum<queue>, error out=w20:errorcluster)  [unwired: 3 in, 1 out]
  n174 = while {
    tunnel: w13 -> [w396]
    tunnel: w20 -> [_]
    stop <- FALSE stop-if-true
    n175 = Get Queue Status(queue=w396) -> (queue out=w393:refnum<queue>, # elements in queue=w392:i32)  [unwired: 2 in, 6 out]
    n176 = Wait (ms)(milliseconds to wait=u32 1000 ("等待时间（毫秒）")) -> ()  [unwired: 1 out]
    n177 = case shown="0" w392 {
      tunnel: w393 -> [_ w423]
      frame Default {
      }
      frame 0 {
        w412 = u16 0 items=["空闲"=0, "水样测试"=1, "标样核查"=2, "零点核查"=3, "跨度核查"=4, "空白测试"=5, "平行样测试"=6, "加标回收"=7, "空白校准"=8, "标样校准"=9, "初始化（清洗）"=10, "调试"=22, "填充管路"=30, "清洗管路"=31, "清洗反应杯"=32] ("工作状态")
        # "试剂填充 172 \n管路清洗108\n氨氮92\n总磷131\n总磷海水147\n总氮76\n总氮海水92"
        n178 = global read "VAR挥发酚全局变量.vi" "状态告警区"() -> (w413:T6)
        n179 = Unbundle By Name(w413) -> ("系统时间"=w419:timestamp, "工作状态"=w411:u16)
        n180 = global read "挥发酚断电保存全局变量.vi" "站号"() -> (w399:u16)
        n181 = Get Date/Time In Seconds() -> (seconds since 1Jan1904=w418:timestamp)
        n182 = Bundle By Name(cluster=cluster{"命令":string, "data":variant} {"命令"="", "data"=variant} ("元素"), "命令"="读状态告警区", "data"=w399) -> (w421:cluster{"命令":string, "data":variant})
        n183 = Equal?(x=w411, y=w412) -> ()  [unwired: 1 out]
        n184 = Subtract(x=w418, y=w419) -> (x-y=w417:dbl)
        n185 = Bundle By Name(cluster=cluster{"命令":string, "data":variant} {"命令"="", "data"=variant} ("元素"), "命令"="读测量数据区", "data"=w399) -> (w407:cluster{"命令":string, "data":variant})
        n186 = Enqueue Element(queue=w423, element=w421) -> (queue out=w405:refnum<queue>)  [unwired: 2 in, 2 out]
        n187 = Absolute Value(x=w417) -> (abs(x)=w416:dbl)
        n188 = global read "VAR挥发酚全局变量.vi" "通讯状态"() -> (w409:bool)
        n189 = Bundle By Name(cluster=cluster{"命令":string, "data":variant} {"命令"="", "data"=variant} ("元素"), "命令"="读关键参数区", "data"=w399) -> (w403:cluster{"命令":string, "data":variant})
        n190 = Enqueue Element(queue=w405, element=w407) -> (queue out=w401:refnum<queue>)  [unwired: 2 in, 2 out]
        n191 = Greater Or Equal?(x=w416, y=30.0) -> (x >= y?=w414:bool)
        n192 = And(x=w414, y=w409) -> (x .and. y?=w410:bool)
        n193 = Enqueue Element(queue=w401, element=w403) -> (queue out=w400:refnum<queue>)  [unwired: 2 in, 2 out]
        n194 = case shown="真" w410 {
          tunnel: w400 -> [_ w428]
          tunnel: w399 -> [_ w426]
          frame False {
          }
          frame True {
            n195 = Bundle By Name(cluster=T16 {"站号"=21, "量程切换"=enum."AUTO", "控制命令"=13, "模式设置"=enum."待机", "测量间隔"=0} ("参数"), "站号"=w426) -> (w424:T16)
            n196 = call "挥发酚启动命令.vi"("参数"=w424) -> ("启动命令"=w427:cluster{"命令":string, "data":variant})  [unwired: 10 in]
            n197 = Enqueue Element(queue=w428, element=w427) -> ()  [unwired: 2 in, 3 out]
          }
        }
      }
    }
    n198 = global read "挥发酚断电保存全局变量.vi" "MB通信方式选择"() -> (w394:enum16{"串口", "TCP"})
    n199 = global read "挥发酚断电保存全局变量.vi" "远程校准量程"() -> (w390:enum16{"低量程1", "低量程2", "高量程1", "高量程2"})
    n200 = global read "挥发酚断电保存全局变量.vi" "远程标样校准"() -> (w391:enum16{"标液1", "标液2", "标液3", "标液4"})
    n201 = local write "平台反控校准量程"(w390) -> ()
    n202 = local write "平台反控标样校准"(w391) -> ()
    n203 = case shown="\"TCP\"" w394 {
      tunnel: [w429 w430] -> w395
      frame "串口", Default {
        n204 = global read "挥发酚断电保存全局变量.vi" "VISA Resource"() -> (w429:refnum<visa-resource-name>)
      }
      frame "TCP" {
        n205 = global read "挥发酚断电保存全局变量.vi" "IP"() -> (w430:string)
      }
    }
    "字符串" <- w395
  }
  n206 = while {
    tunnel: w13 -> [w433]
    tunnel: w15 -> [w432]
    tunnel: w9 -> [w431]
    stop <- FALSE stop-if-true
    n207 = event shown="[4] \"手动启动\": 值改变" {
      selector: _ -> [_ _ _ _ _ _ _ _]
      dyn-events: _ -> [_ _ _ _ _ _ _ _]
      timeout: _ -> [_ _ _ _ _ _ _ _]
      tunnel: w433 -> [_ _ _ _ w448 w463 _ _]
      tunnel: w432 -> [_ _ _ _ _ w465 _ _]
      tunnel: w431 -> [_ _ _ _ _ _ w468 _]
      event Timeout {
        n208 = event-data() -> ()  [unwired: 1 in, 3 out]
      }
      event "布尔": Value Change {
        n209 = event-data() -> ("NewVal"=w435:bool)  [unwired: 1 in, 5 out]
        n210 = case shown="假" w435 {
          frame False {
            n211 = global write "VAR挥发酚全局变量.vi" "权限等级"(enum16{"一级权限", "二级权限", "三级权限", "超级权限"}."一级权限" ("权限等级")) -> ()
          }
          frame True {
            n212 = global read "VAR挥发酚全局变量.vi" "权限密码"() -> (w439:u32[])
            n213 = global read "VAR挥发酚全局变量.vi" "权限等级"() -> (w438:enum16{"一级权限", "二级权限", "三级权限", "超级权限"})
            n214 = call "密码权限设置.vi"("权限输入"=w438, "权限密码"=w439) -> ("权限输出"=w437:enum16{"一级权限", "二级权限", "三级权限", "超级权限"})  [unwired: 9 in]
            n215 = global write "VAR挥发酚全局变量.vi" "权限等级"(w437) -> ()
          }
        }
      }
      event "权限等级": Mouse Down {
        n216 = event-data() -> ()  [unwired: 1 in, 8 out]
        n217 = global read "VAR挥发酚全局变量.vi" "权限密码"() -> (w442:u32[])
        n218 = global read "VAR挥发酚全局变量.vi" "权限等级"() -> (w441:enum16{"一级权限", "二级权限", "三级权限", "超级权限"})
        n219 = call "密码权限设置.vi"("权限输入"=w441, "权限密码"=w442) -> ("权限输出"=w440:enum16{"一级权限", "二级权限", "三级权限", "超级权限"})  [unwired: 9 in]
        n220 = global write "VAR挥发酚全局变量.vi" "权限等级"(w440) -> ()
      }
      event "平台反控校准量程", "平台反控标样校准": Value Change {
        n221 = event-data() -> ()  [unwired: 1 in, 6 out]
        n222 = flat-sequence {
          frame #0 {
            n223 = global write "挥发酚断电保存全局变量.vi" "远程校准量程"("平台反控校准量程") -> ()
            n224 = global write "挥发酚断电保存全局变量.vi" "远程标样校准"("平台反控标样校准") -> ()
          }
          frame #1 {
            n225 = call "配置文件保存.vi"() -> ()  [unwired: 12 in]
          }
        }
      }
      event "手动启动": Value Change {
        n226 = event-data() -> ()  [unwired: 1 in, 6 out]
        n227 = call "挥发酚启动参数对话框.vi"() -> ("标样浓度输出"=w446:dbl, "确认"=w445:bool, "元素"=w447:cluster{"命令":string, "data":variant})  [unwired: 9 in]
        n228 = case shown="真" w445 {
          tunnel: w448 -> [_ w457]
          tunnel: w447 -> [_ w456]
          tunnel: w446 -> [_ w451]
          frame False {
          }
          frame True {
            (unwired) u16 31 ("y")
            n229 = Enqueue Element(queue=w457, element=w456) -> ()  [unwired: 2 in, 3 out]
            n230 = global write "VAR挥发酚全局变量.vi" "手动启动"(TRUE ("手动启动")) -> ()
            n231 = Unbundle By Name(w456) -> ("data"=w455:variant)
            n232 = Variant To Data(type=cluster{"站号":u16, "控制命令":u16[]} {"站号"=0, "控制命令"=[]} ("输出簇"), Variant=w455) -> (data=w453:cluster{"站号":u16, "控制命令":u16[]})  [unwired: 1 in, 1 out]
            n233 = Unbundle By Name(w453) -> ("控制命令"=w452:u16[])
            n234 = Index Array(array=w452) -> (element=w449:u16)  [unwired: 1 in]
            n235 = case shown="0, 默认" w449 {
              tunnel: w451 -> [_ w458]
              frame 0, Default {
              }
              frame 2 {
                # "标样核查"
                n236 = flat-sequence {
                  tunnel: w458 -> [w459]
                  frame #0 {
                    n237 = global read "挥发酚断电保存全局变量.vi" "质控参数设置"() -> (w461:T17)
                    n238 = Bundle By Name(cluster=w461, "标准液标准浓度"=w459) -> (w460:T17)
                    n239 = global write "挥发酚断电保存全局变量.vi" "质控参数设置"(w460) -> ()
                  }
                  frame #1 {
                    n240 = call "配置文件保存.vi"() -> ()  [unwired: 12 in]
                  }
                }
              }
            }
          }
        }
      }
      event "停止": Value Change {
        n241 = event-data() -> ()  [unwired: 1 in, 6 out]
        n242 = Cancel Notification(0:w465) -> (8:w466:refnum<notifier>)  [unwired: 1 in, 2 out]
        n243 = Send Notification(notification=TRUE ("通知"), notifier=w466) -> ()  [unwired: 1 in, 2 out]
        n244 = Enqueue Element(queue=w463, element=cluster{"命令":string, "data":variant} {"命令"="启动", "data"=variant(cluster{"站号":u16, u16[]} {"站号"=1, [11]})} ("元素")) -> ()  [unwired: 2 in, 3 out]
      }
      event "设置", "参数查询": Value Change {
        n245 = event-data() -> ()  [unwired: 1 in, 6 out]
        n246 = invoke on="子面板" class="SubPnl" method="Remove VI"() -> (error out=w469:errorcluster)  [unwired: 3 in, 2 out]
        n247 = property on="窗格" class="Pane"("Origin"=T4 {"Horizontal"=0, "Vertical"=628} ("原点")) -> ()  [unwired: 2 in, 2 out]
        n248 = invoke on="子面板" class="SubPnl" method="Insert VI"(error in=w469, "VI Ref"=w468) -> ()  [unwired: 2 in, 4 out]
        n249 = global write "VAR挥发酚全局变量.vi" "页面"(enum16{"主页", "参数页", "校准页"}."参数页" ("页面")) -> ()
      }
      event "返回", "返回 2", "返回 3": Value Change {
        n250 = event-data() -> ()  [unwired: 1 in, 6 out]
        n251 = global write "VAR挥发酚全局变量.vi" "页面"(enum16{"主页", "参数页", "校准页"}."主页" ("页面")) -> ()
        n252 = property on="窗格" class="Pane"("Origin"=T4 {"Horizontal"=0, "Vertical"=0} ("原点")) -> ()  [unwired: 2 in, 2 out]
      }
    }
  }
  n253 = call "Close TimingControl.vi"("error in (no error)"=w1, "TimingControl in"=w2) -> ()  [unwired: 9 in, 1 out]
